vi "AcquireWaveforms.vi.vi"(8 "error in (no error)":errorcluster, 11 "923x Acquisition Config":T1={"Acq"=FALSE, "NumberOfModules"=0, "Dynamic FPGA VI Ref"=refnum, "KeyphasorX3"=[], "FixedSizeX32"={"EnabledChannels"=[], "Sensitivity"=[], "InputConfig"=[]}, "SamplingInfo"={"Number of Channels"=4, "Sampling Rate"=4.0, "Channels"=[], "Units"=[], "Offsets"=[]}, "Normal Mode Sample Rate"=0.0, "BlockSize (sec)"=0.0, "Samples To Read (per chan)"=0, "RunningAcquisitionLength"=0.0, "Settling Time"=0.0, "Fpga Tach Buffer Size (samples)"=0, "Waveform Groups"=[], "Acquisition Block Number"=0, "Device Name"="", "ValidConfig"=FALSE, "Last Dynamic Module"="", "HighPassFilterState"=[], "Low Frequency Cutoff"=[], "BurstMode"={"Acquisition Time"=0.0, "Sample Rate"=0.0, "Collection Reason"=""}, "DAQ task"=""} {"HighPassFilterState"."Filter State" format="%.2f"; "HighPassFilterState"."IIR Filter Cluster"."Forward Coefficients" format="%.2f"; "HighPassFilterState"."IIR Filter Cluster"."Reverse Coefficients" format="%.2f"; "FixedSizeX32"."InputConfig" items=["AC Coupled", "DC Coupled", "IEPE AC Coupled"]}) -> (0 "error out":errorcluster, 3 "Waveforms":waveform(sgl)[](array[waveform]))   [LabVIEW 2017, in "TSNcDAQ_AI.lvlib"]
uses:
  <vilib>/addons/InsightCM/Devices/Shared/Cms/DAQmx/TSNcDAQ_AI.lvlib
  <vilib>/addons/InsightCM/Devices/Shared/Cms/CmsAcquisition/controls/Configuration.ctl
  <vilib>/addons/InsightCM/Devices/Shared/Cms/CmsAcquisition/controls/TachometerConfig.ctl
  <vilib>/addons/InsightCM/Devices/Shared/Cms/CmsAcquisition/controls/FixedSizeArrays.ctl
  <vilib>/LabVIEW Targets/FPGA/cRIO/shared/nicrio_ModuleControls/nicrio_cRIO-9232_ConfigModeRing.ctl
  <vilib>/addons/InsightCM/Devices/Shared/Cms/cRIOWfmAcq/subVIs/RIO Wfm Cust Ctrls/rwfm_SamplingInfo.ctl
  <vilib>/addons/InsightCM/Devices/Shared/Cms/CmsAcquisition/controls/Group.ctl
  <vilib>/addons/InsightCM/Devices/Shared/Cms/CmsAcquisition/controls/Channel.ctl
  <vilib>/addons/InsightCM/Utilities/Analysis/Vibration/controls/HighPassFilterState.ctl
  <vilib>/addons/InsightCM/Devices/Shared/Cms/CmsAcquisition/controls/BurstMode.ctl
  <vilib>/DAQmx/read.llb/DAQmx Read (Analog 1D Wfm NChan NSamp).vi
  <vilib>/DAQmx/miscellaneous.llb/DAQmx Fill In Error Info.vi
  <vilib>/addons/InsightCM/Utilities/ChannelStatus/ChannelStatus.lvlib
  <vilib>/addons/InsightCM/Utilities/Analysis/Vibration/VibrationAnalysisFunctions.lvlib
  <vilib>/addons/InsightCM/Devices/Shared/Cms/CmsAcquisition/CmsAcquisition.lvlib
  <vilib>/addons/InsightCM/Devices/Shared/Cms/cRIOWfmAcq/cRIOWfmLib.lvlib
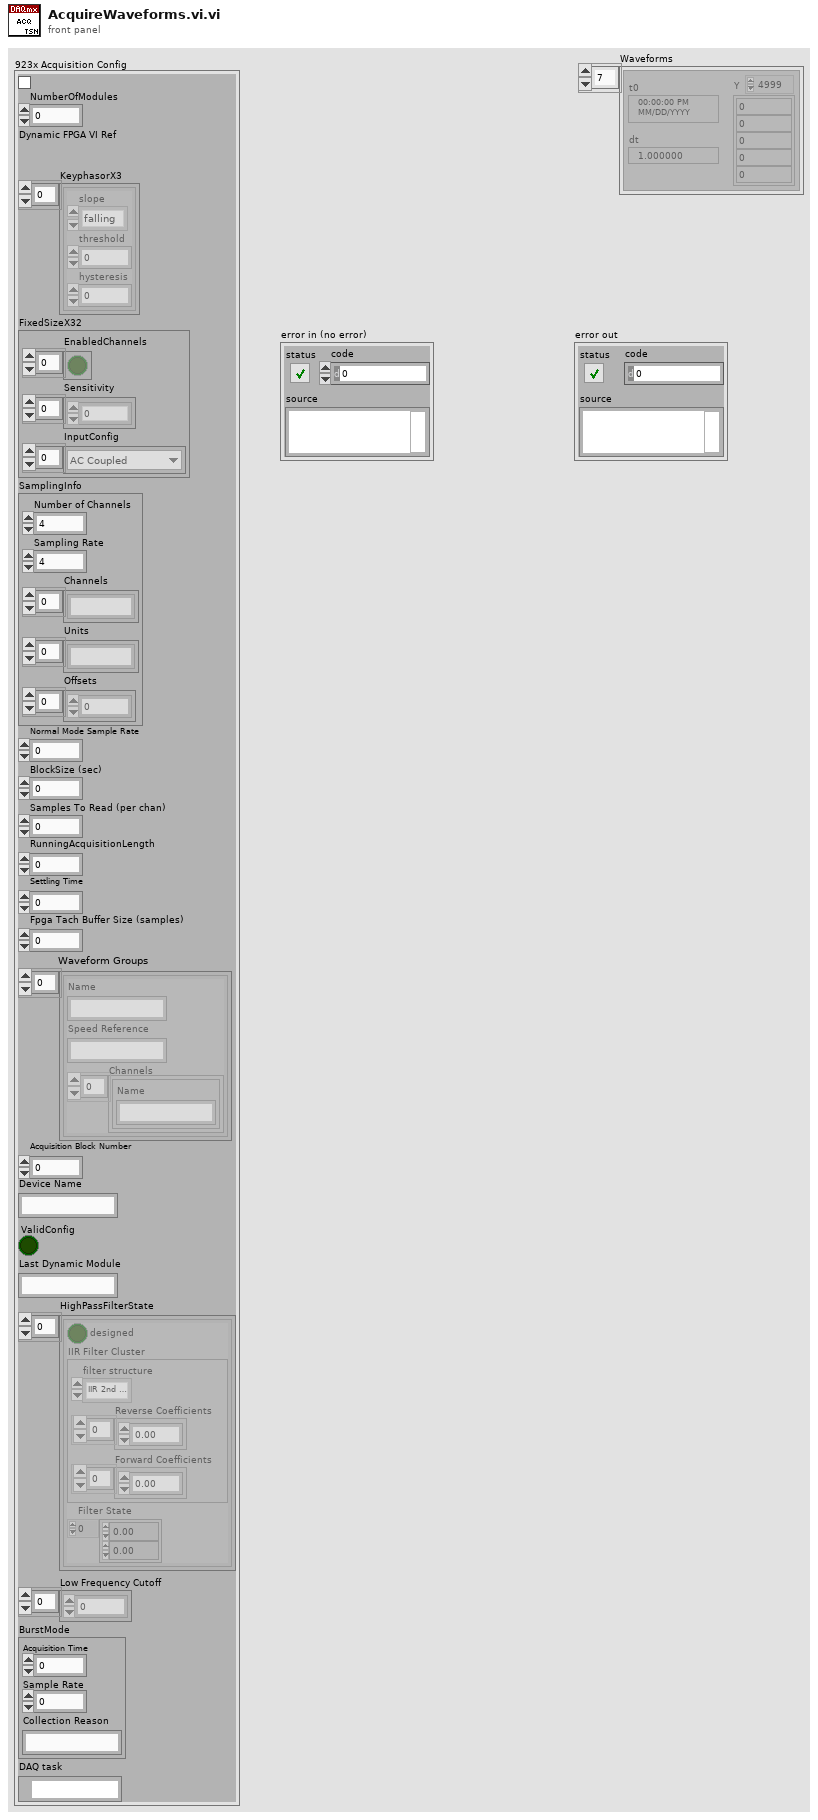
[diagram p1: front panel]
types:
  T1 = typedef "CmsAcquisition.lvlib/Configuration.ctl" = cluster{"Acq":bool, "NumberOfModules":i16, "Dynamic FPGA VI Ref":refnum<k20>, "KeyphasorX3":T2[], "FixedSizeX32":T3, "SamplingInfo":T5, "Normal Mode Sample Rate":dbl, "BlockSize (sec)":dbl, "Samples To Read (per chan)":i32, "RunningAcquisitionLength":dbl, "Settling Time":dbl, "Fpga Tach Buffer Size (samples)":i32, "Waveform Groups":T6[], "Acquisition Block Number":i32, "Device Name":string, "ValidConfig":bool, "Last Dynamic Module":string, "HighPassFilterState":T8[], "Low Frequency Cutoff":dbl[], "BurstMode":T9, "DAQ task":refnum<k21>}
  T2 = typedef "CmsAcquisition.lvlib/TachometerConfig.ctl" = cluster{"slope":enum16{"falling", "rising"}, "threshold":dbl, "hysteresis":dbl}
  T3 = typedef "CmsAcquisition.lvlib/FixedSizeArrays.ctl" = cluster{"EnabledChannels":bool[], "Sensitivity":dbl[], "InputConfig":T4[]}
  T4 = typedef "nicrio_cRIO-9232_ConfigModeRing.ctl" = u8
  T5 = typedef "cRIOWfmLib.lvlib/rwfm_SamplingInfo.ctl" = cluster{"Number of Channels":i32, "Sampling Rate":dbl, "Channels":string[], "Units":string[], "Offsets":sgl[]}
  T6 = typedef "CmsAcquisition.lvlib/Group.ctl" = cluster{"Name":string, "Speed Reference":string, "Channels":T7[]}
  T7 = typedef "CmsAcquisition.lvlib/Channel.ctl" = cluster{"Name":string}
  T8 = typedef "VibrationAnalysisFunctions.lvlib/HighPassFilterState.ctl" = cluster{"designed":bool, "IIR Filter Cluster":cluster{"filter structure":enum32{"IIR 2nd Order", "IIR 4th Order"}, "Reverse Coefficients":dbl[], "Forward Coefficients":dbl[]}, "Filter State":dbl[]}
  T9 = typedef "CmsAcquisition.lvlib/BurstMode.ctl" = cluster{"Acquisition Time":dbl, "Sample Rate":dbl, "Collection Reason":string}
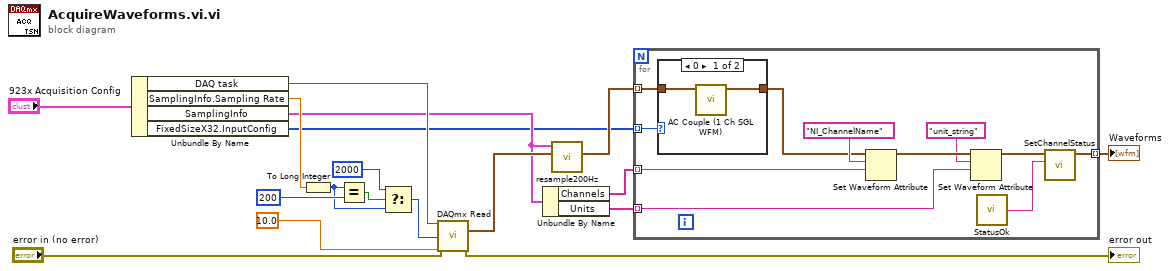
[diagram p0: block diagram]
diagram:
  n1 = Unbundle By Name("923x Acquisition Config") -> ("DAQ task"=w13:refnum<k21>, "SamplingInfo.Sampling Rate"=w16:dbl, "SamplingInfo"=w4:T5, "FixedSizeX32.InputConfig"=w1:T4[])
  n2 = To Long Integer(number=w16) -> (32bit integer=w8:i32)
  n3 = Equal?(x=w8, y=200) -> (x = y?=w10:bool)
  n4 = Select(t=2000 ("y"), s=w10, f=w8) -> (s? t:f=w7:i32)
  n5 = call-poly <vilib>:"DAQmx Read.vi"("task/channels in"=w13, "number of samples per channel"=w7, "timeout"=10.0, "error in"="error in (no error)") -> ("data"=w12:waveform(dbl)[], "error out"=→"error out":errorcluster)  [unwired: 9 in, 1 out]
  n6 = Unbundle By Name(w4) -> ("Channels"=w3:string[], "Units"=w2:string[])
  n7 = call <vilib>:"resample200Hz.vi"("Original Waveforms"=w12, "SamplingInfo"=w4) -> ("Resampled Waveforms"=w6:waveform(sgl)[])  [unwired: 9 in]
  n8 = for {
    tunnel: w6 -> [w20] mode=indexing
    tunnel: [w24] -> w5 mode=indexing
    tunnel: w3 -> [w23] mode=indexing
    tunnel: w2 -> [w22] mode=indexing
    tunnel: w1 -> [w21] mode=indexing
    n9 = case shown="0" w21 {
      tunnel: w20 -> [w31 w32]
      tunnel: [w30 w32] -> w19
      frame 0 {
        n10 = call <vilib>:"AC Couple (1 Ch SGL WFM).vi"("Signal"=w31) -> ("AC Coupled"=w30:waveform(sgl))  [unwired: 8 in, 2 out]
      }
      frame 1, Default {
      }
    }
    n11 = Set Waveform Attribute(5:w23, 6:"NI_ChannelName" ("name"), 7:w19) -> (3:w29:waveform(sgl))  [unwired: 1 in, 2 out]
    n12 = Set Waveform Attribute(5:w22, 6:"unit_string" ("name"), 7:w29) -> (3:w25:waveform(sgl))  [unwired: 1 in, 2 out]
    n13 = call <vilib>:"StatusOk.vi"() -> ("status"=w26:string)  [unwired: 5 in]
    n14 = call <vilib>:"SetChannelStatus.vi"("Channel Status"=w26, "Waveform in"=w25) -> ("Waveform out"=w24:waveform(sgl))  [unwired: 8 in, 1 out]
  }
  "Waveforms" <- w5
